vi "Configure Frequency (Center Span).vi"(8 "error in (no error)":errorcluster, 9 "Span (2.65E+10 Hz)":dbl=26500000000.0, 10 "Center Frequency (1.325E+10 Hz)":dbl=13250000000.0 format="%#.6g", 11 "VISA resource name":refnum<visa-resource-name>) -> (0 "error out":errorcluster, 3 "VISA resource name out":refnum<visa-resource-name>)   [LabVIEW 2018, in "Agilent MXA Series.lvlib"]
doc: "Configures the frequency range of the spectrum analyzer using the center frequency and the frequency span. If span corresponds to zero Hertz, then the spectrum analyzer operates in time-domain mode. Otherwise, spectrum analyzer operates in frequency-domain mode.\n\n Frequency Start = Center Frequency - Span/2\n Frequency Stop = Center Frequency + Span/2"
uses:
  Agilent MXA Series.lvlib
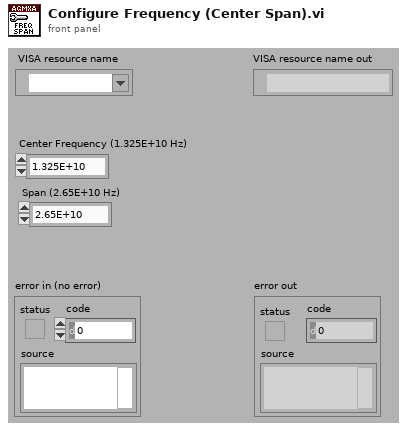
[diagram p1: front panel]
types:
  T1 = typedef "Agilent MXA Series.lvlib/Extended User Data.ctl" = cluster{"Measurement Type":i32, "Agilent MXA/EXA Model":i32}
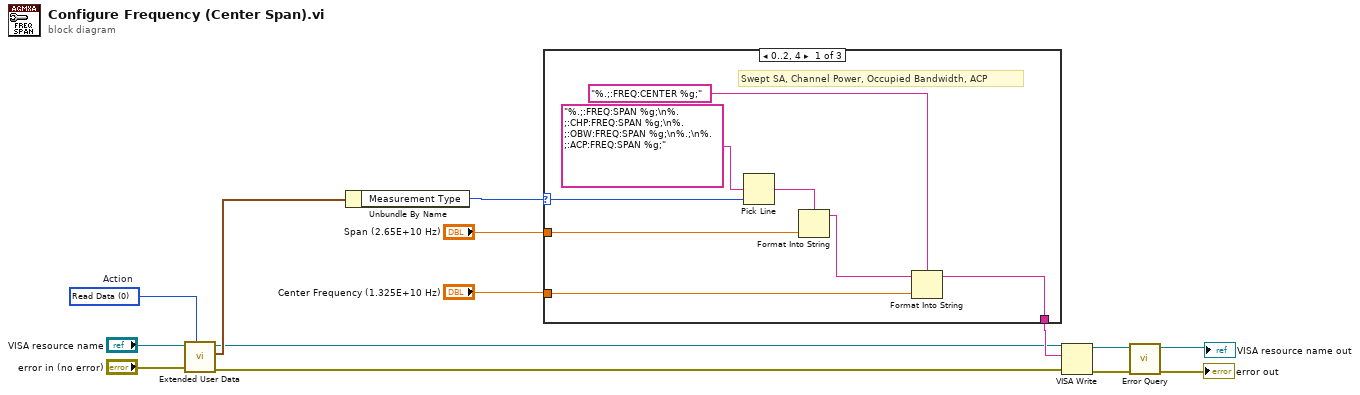
[diagram p0: block diagram]
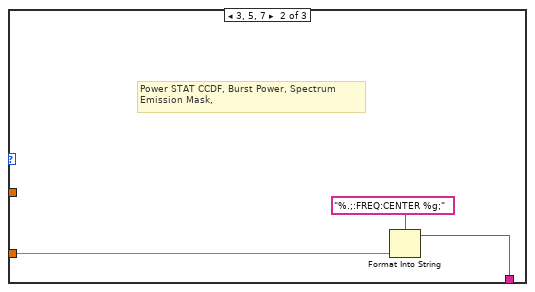
[diagram p2: hidden frame]
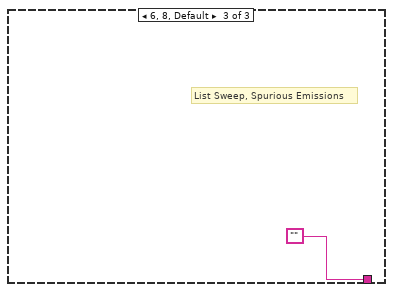
[diagram p3: hidden frame]
diagram:
  w1 = 0 items=["Read Data", "Write Data", "Clear Data", "Clear ALL Data"]  # Action
  n1 = call "Extended User Data.vi"("Action (1:Write Data)"=w1, "Error In (no error)"="error in (no error)", "VISA resource name in"="VISA resource name") -> ("Error Out"=w6:errorcluster, "User Data Out"=w11:T1, "VISA resource name out"=w7:refnum<visa-resource-name>)  [unwired: 6 in]
  n2 = Unbundle By Name(w11) -> ("Measurement Type"=w8:i32)
  n3 = case shown="0..2, 4" w8 {
    selector: w8 -> [w21 _ _]
    tunnel: "Span (2.65E+10 Hz)" -> [w19 _ _]
    tunnel: "Center Frequency (1.325E+10 Hz)" -> [w16 w24 _]
    tunnel: [w15 w23 ""] -> w14
    frame 0..2, 4 {
      # "Swept SA, Channel Power, Occupied Bandwidth, ACP"
      n4 = Pick Line(multi-line string="%.;:FREQ:SPAN %g;\n%.;:CHP:FREQ:SPAN %g;\n%.;:OBW:FREQ:SPAN %g;\n%.;\n%.;:ACP:FREQ:SPAN %g;", line index=w21) -> (output string=w20:string)  [unwired: 1 in]
      n5 = Format Into String(format string=w20, w19) -> (resulting string=w17:string)  [unwired: 2 in, 1 out]
      n6 = Format Into String(format string="%.;:FREQ:CENTER %g;", initial string=w17, w16) -> (resulting string=w15:string)  [unwired: 1 in, 1 out]
    }
    frame 3, 5, 7 {
      # "Power STAT CCDF, Burst Power, Spectrum \nEmission Mask,"
      n7 = Format Into String(format string="%.;:FREQ:CENTER %g;", w24) -> (resulting string=w23:string)  [unwired: 2 in, 1 out]
    }
    frame 6, 8, Default {
      # "List Sweep, Spurious Emissions"
    }
  }
  n8 = VISA Write(VISA resource name=w7, write buffer=w14, error in (no error)=w6) -> (VISA resource name out=w5:refnum<visa-resource-name>, error out=w4:errorcluster)  [unwired: 1 out]
  n9 = call "Error Query.vi"("error in (no error)"=w4, "VISA resource name"=w5) -> ("error out"=→"error out":errorcluster, "VISA resource name out"=→"VISA resource name out":refnum<visa-resource-name>)  [unwired: 6 in, 2 out]
